vi "checkForceErrorInRange.vi"(8 "error in (no error)":errorcluster, 11 "SystemController in":refnum<class "SystemController.lvclass">) -> (0 "error out":errorcluster, 2 "forceErrorInRangeIsTrue":bool, 3 "SystemController out":refnum<class "SystemController.lvclass">)   [LabVIEW 2015]
uses:
  SystemController.lvclass
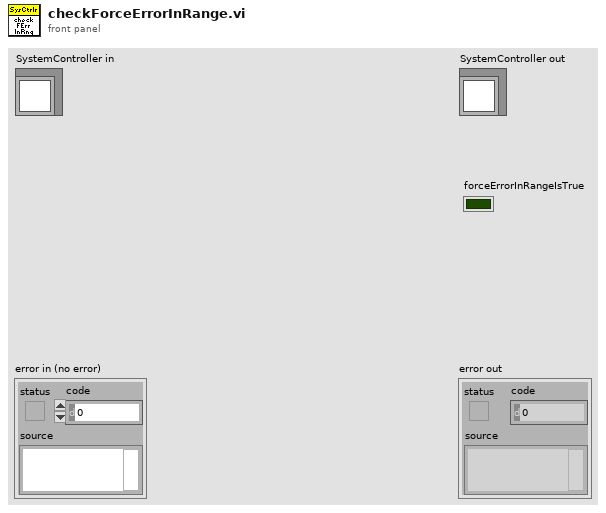
[diagram p1: front panel]
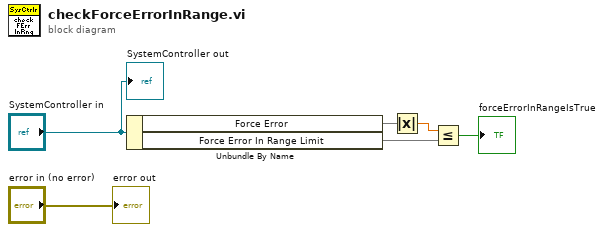
[diagram p0: block diagram]
diagram:
  n1 = Unbundle By Name("SystemController in") -> ("Force Error"=w4, "Force Error In Range Limit"=w3)
  n2 = Absolute Value(x=w4) -> (abs(x)=w2:dbl)
  n3 = Less Or Equal?(x=w2, y=w3) -> (x <= y?=→"forceErrorInRangeIsTrue":bool)
  "error out" <- "error in (no error)"
  "SystemController out" <- "SystemController in"
